vi "Host Approach RetractionA1.vi"() -> ()   [LabVIEW 2012]
uses:
  <vilib>/FPGAPlugInAG/PCI-7831R/niLvFpga_Open_PCI-7831R.vi
  <vilib>/rvi/interface/common/dynamic/niFpgaDynamicAddResources.vi
  <vilib>/Utility/error.llb/Error Cluster From Error Code.vi
  <vilib>/rvi/errors/niLvFpgaAdjustHostInterfaceError.vi
  <vilib>/FPGAPlugInAG/Dynamic/niLvFpga_Close_Dynamic.vi
  <vilib>/FPGAPlugInAG/Dynamic/niLvFpga_Run_Dynamic.vi
  <vilib>/Utility/file.llb/Write To Spreadsheet File (I64).vi
  <vilib>/rvi/interface/nirviOpenFPGA/nirviOpenFPGA.xnode
  SB130-XPS/Documents/FPGA-project-apporach-retraction/FPGA Bitfiles/Apporach-Retract_FPGATarget2_FPGATargetApproa_sPWXUlF8ZuM.lvbitx
  FPGA Target Approach RetractionA2copyAidanV2.vi
  <vilib>/rvi/interface/nirviReadWriteControl/nirviReadWriteControl.xnode
  <vilib>/rvi/interface/nirviCloseFPGA/nirviCloseFPGA.xnode
  <vilib>/rvi/interface/nirviMethod/nirviMethod.xnode
  <vilib>/rvi/interface/Simulation/niFpgaSimulationCallBeginRW.vi
  <vilib>/rvi/errors/niLvFpgaMergeErrorWithErrorCode.vi
  NiFpgaLv.dll
  <vilib>/FPGAPlugInAG/Dynamic/niLvFpga_StartFifo_Dynamic.vi
  <vilib>/FPGAPlugInAG/Dynamic/niLvFpga_StopFifo_Dynamic.vi
  <vilib>/FPGAPlugInAG/Dynamic/niLvFpga_ReadFifo_Dynamic.vi
panel:
  in  "% in for Fast Offset":dbl
  in  "% in for setpoint":dbl
  in  "TF \"Zero\" Point":i16
  out "Bottom Sensor Phase Data":i16[](array[numeric])
  in  "Stop Fine Retraction and start next approach":bool
  in  "Set distance for Bounce or\nretract until TF signal is equal\nto TF in Air":bool
  in  "Bounce Distance (nm)":u32
  out "Fine":i16[](array[numeric])
  out "Course":i16[](array[numeric])
  out "Counter Indicator 2":fxp<+/-,64,32>
  out "fine indicator":i16
  out "TF Phase Data":i16[](graph)
  out "Fine output":i16[](array[numeric])
  out "Course Output":fxp<+/-,64,32>[](array[numeric])
  out "TF Phase data":i16[](array[numeric])
  out "Current Image":u8
  in  "Total Number of Images":u8=1 min=1
  out "step counter":i16
  in  "base path":path=path "C:/Users/Rodolfo/Documents/LAB/2013-05-16-SPM-data"
  in  "file-Name":string="approach-15a"
  in  "Store Data":bool
  out "Bottom Sensor":i16[](graph)
  out "Bottom Sensor \nData":i16[](array[numeric])
  out "Position Data":i16[](array[numeric])
  out "tuning fork amplitude data":i16[](array[numeric])
  in  "Approach Minimum":i32=20000
  out "Approach Setpoint":i32=23000
  out "Fast Approach Offset":i32=29000
  in  "TF in Air":i32=36000
  out "Fine A bits/us":dbl=5.463300000000001e-06
  out "Fine R bits/us":dbl=5.463300000000001e-06
  in  "Fine Approach (nm/s)":dbl=5.0
  in  "Fine Retraction (nm/s)":dbl=5.0
  out "Approach done and fully retracted":bool
  in  "DAQ Rate":i32=8000
  in  "Number of Elements":i32=100
  out "BottomSensor Phase":i16[](graph)
  out "Tuning Fork":i16[](graph)
  out "Fast A nm/s indicator":dbl=200.0
  out "Fast A bits/us":dbl=0.00021853200000000001
  out "Fast R nm/s indicator":dbl=200.0
  out "Fast R bits/us":dbl=0.00021853200000000001
  in  "Fast Approach (nm/s)":dbl=200.0
  in  "Fast Retraction (nm/s)":dbl=200.0
  in  "Automated Approach Start":bool
  out "Numeric":i32=-14468
  out "Counter Indicator":dbl[](graph)
  out "Z Indicator":i16[](graph)
  in  "MCL Counter":i64=100
  in  "MCL Divisions":i32=200
  out "MCL Range Indicator":bool
  out "Host Counter Indicator":i64=115
  out "Digital Steps per Region":i32=327
  out "Host Counter Output":i32=4878
  in  "Z Position MCL Fine":i32
  out "Host Z Position Indicator":i32
  out "Z Position Range Indicator":bool
  out "Z Fine Steps per Region":dbl=0.0049897001602197295
  out "Host Z Output":fxp<+/-,40,30>
  in  "Manual Approach Start":bool
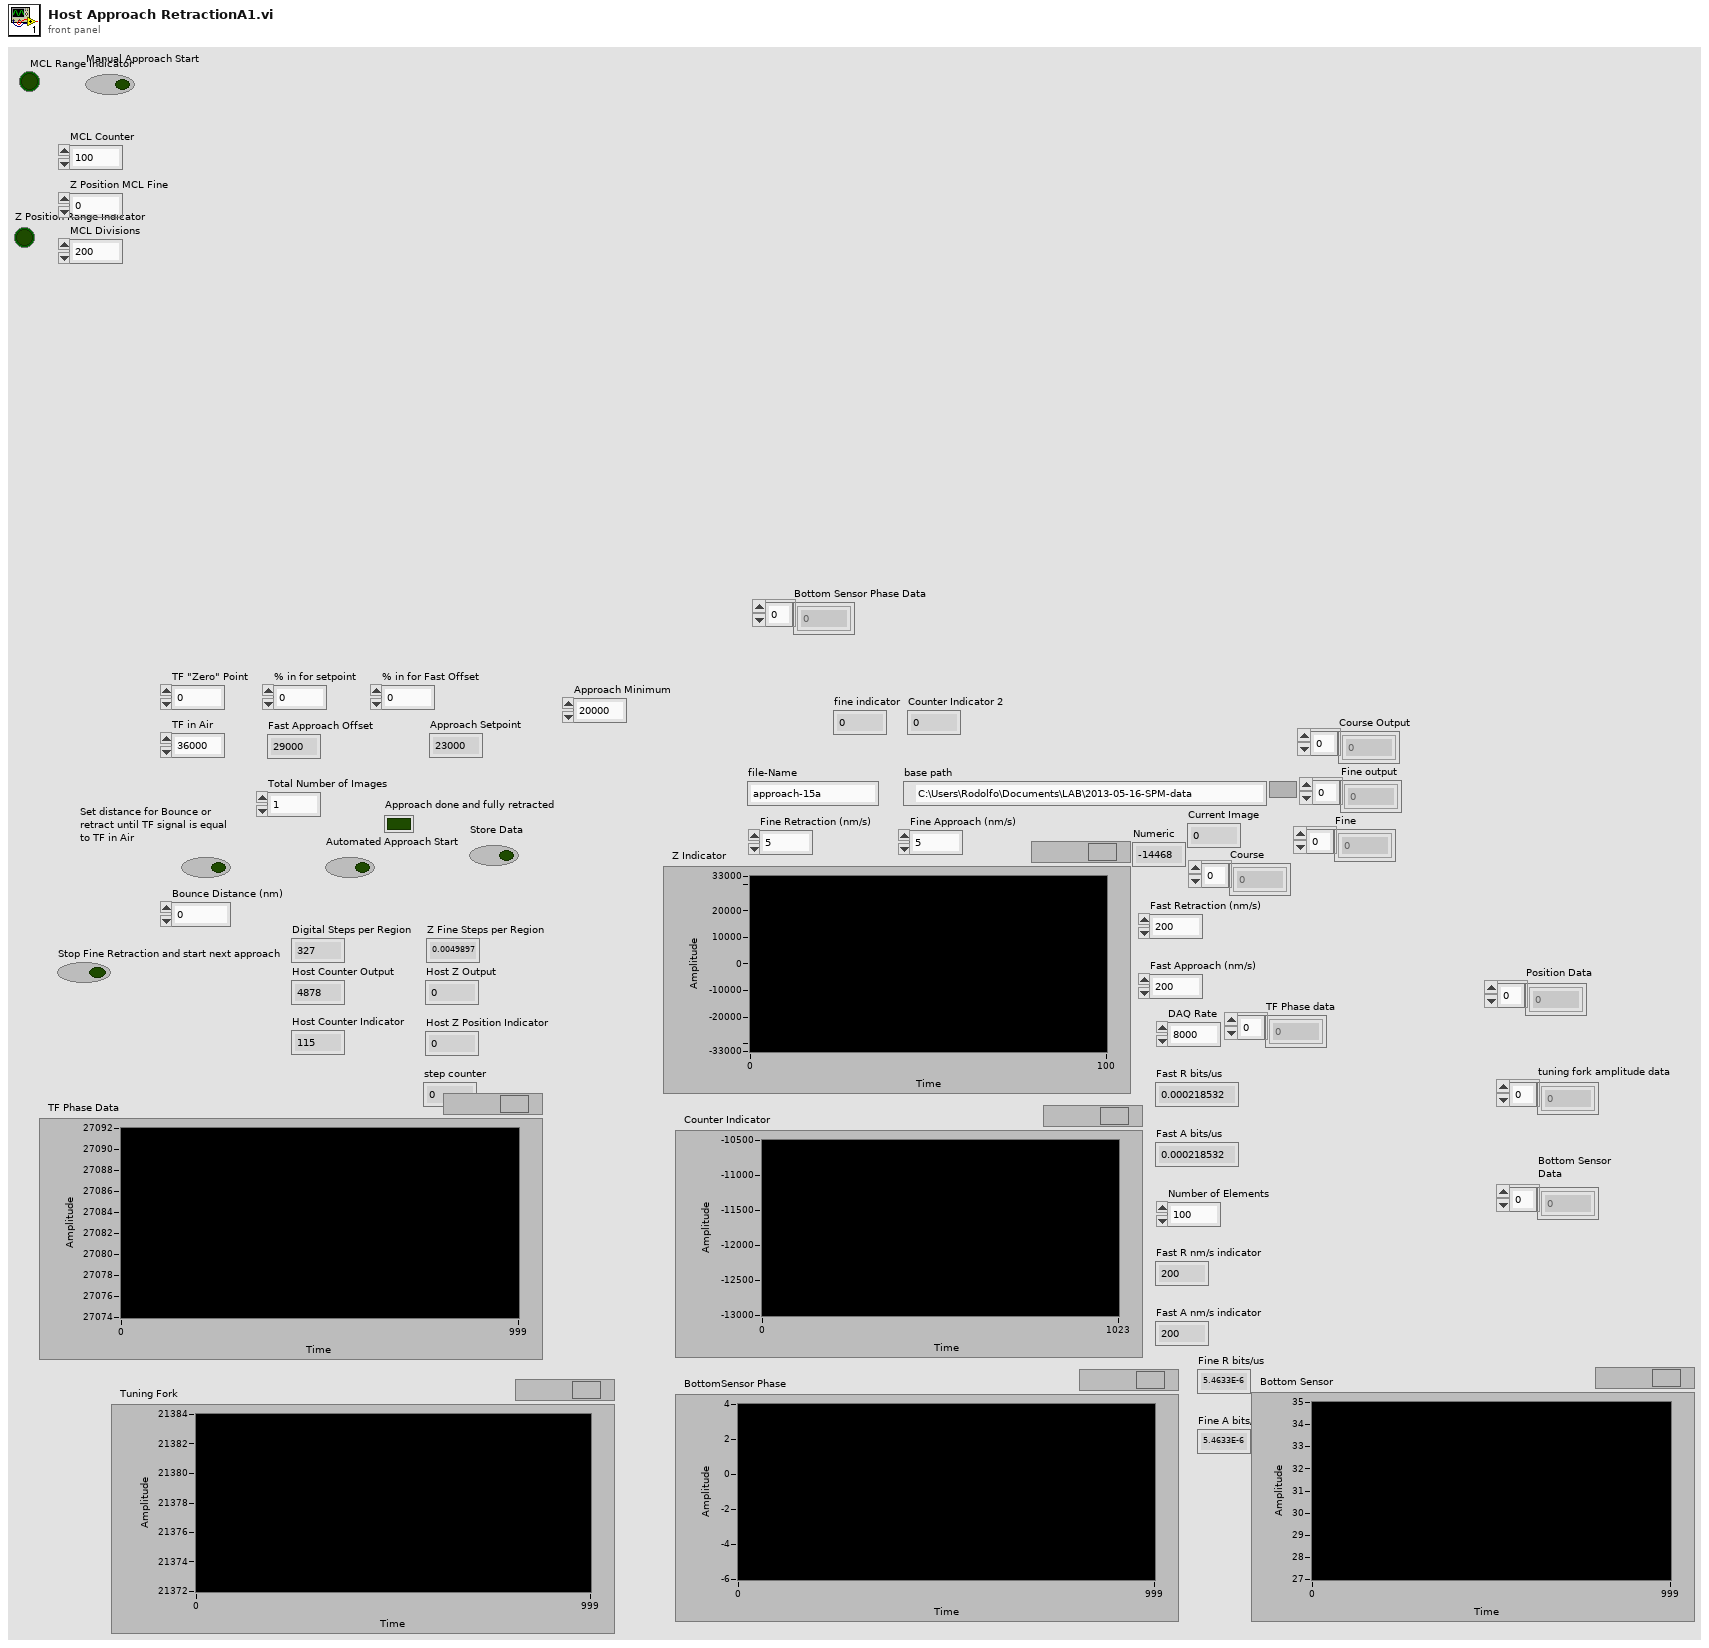
[diagram p1: front panel]
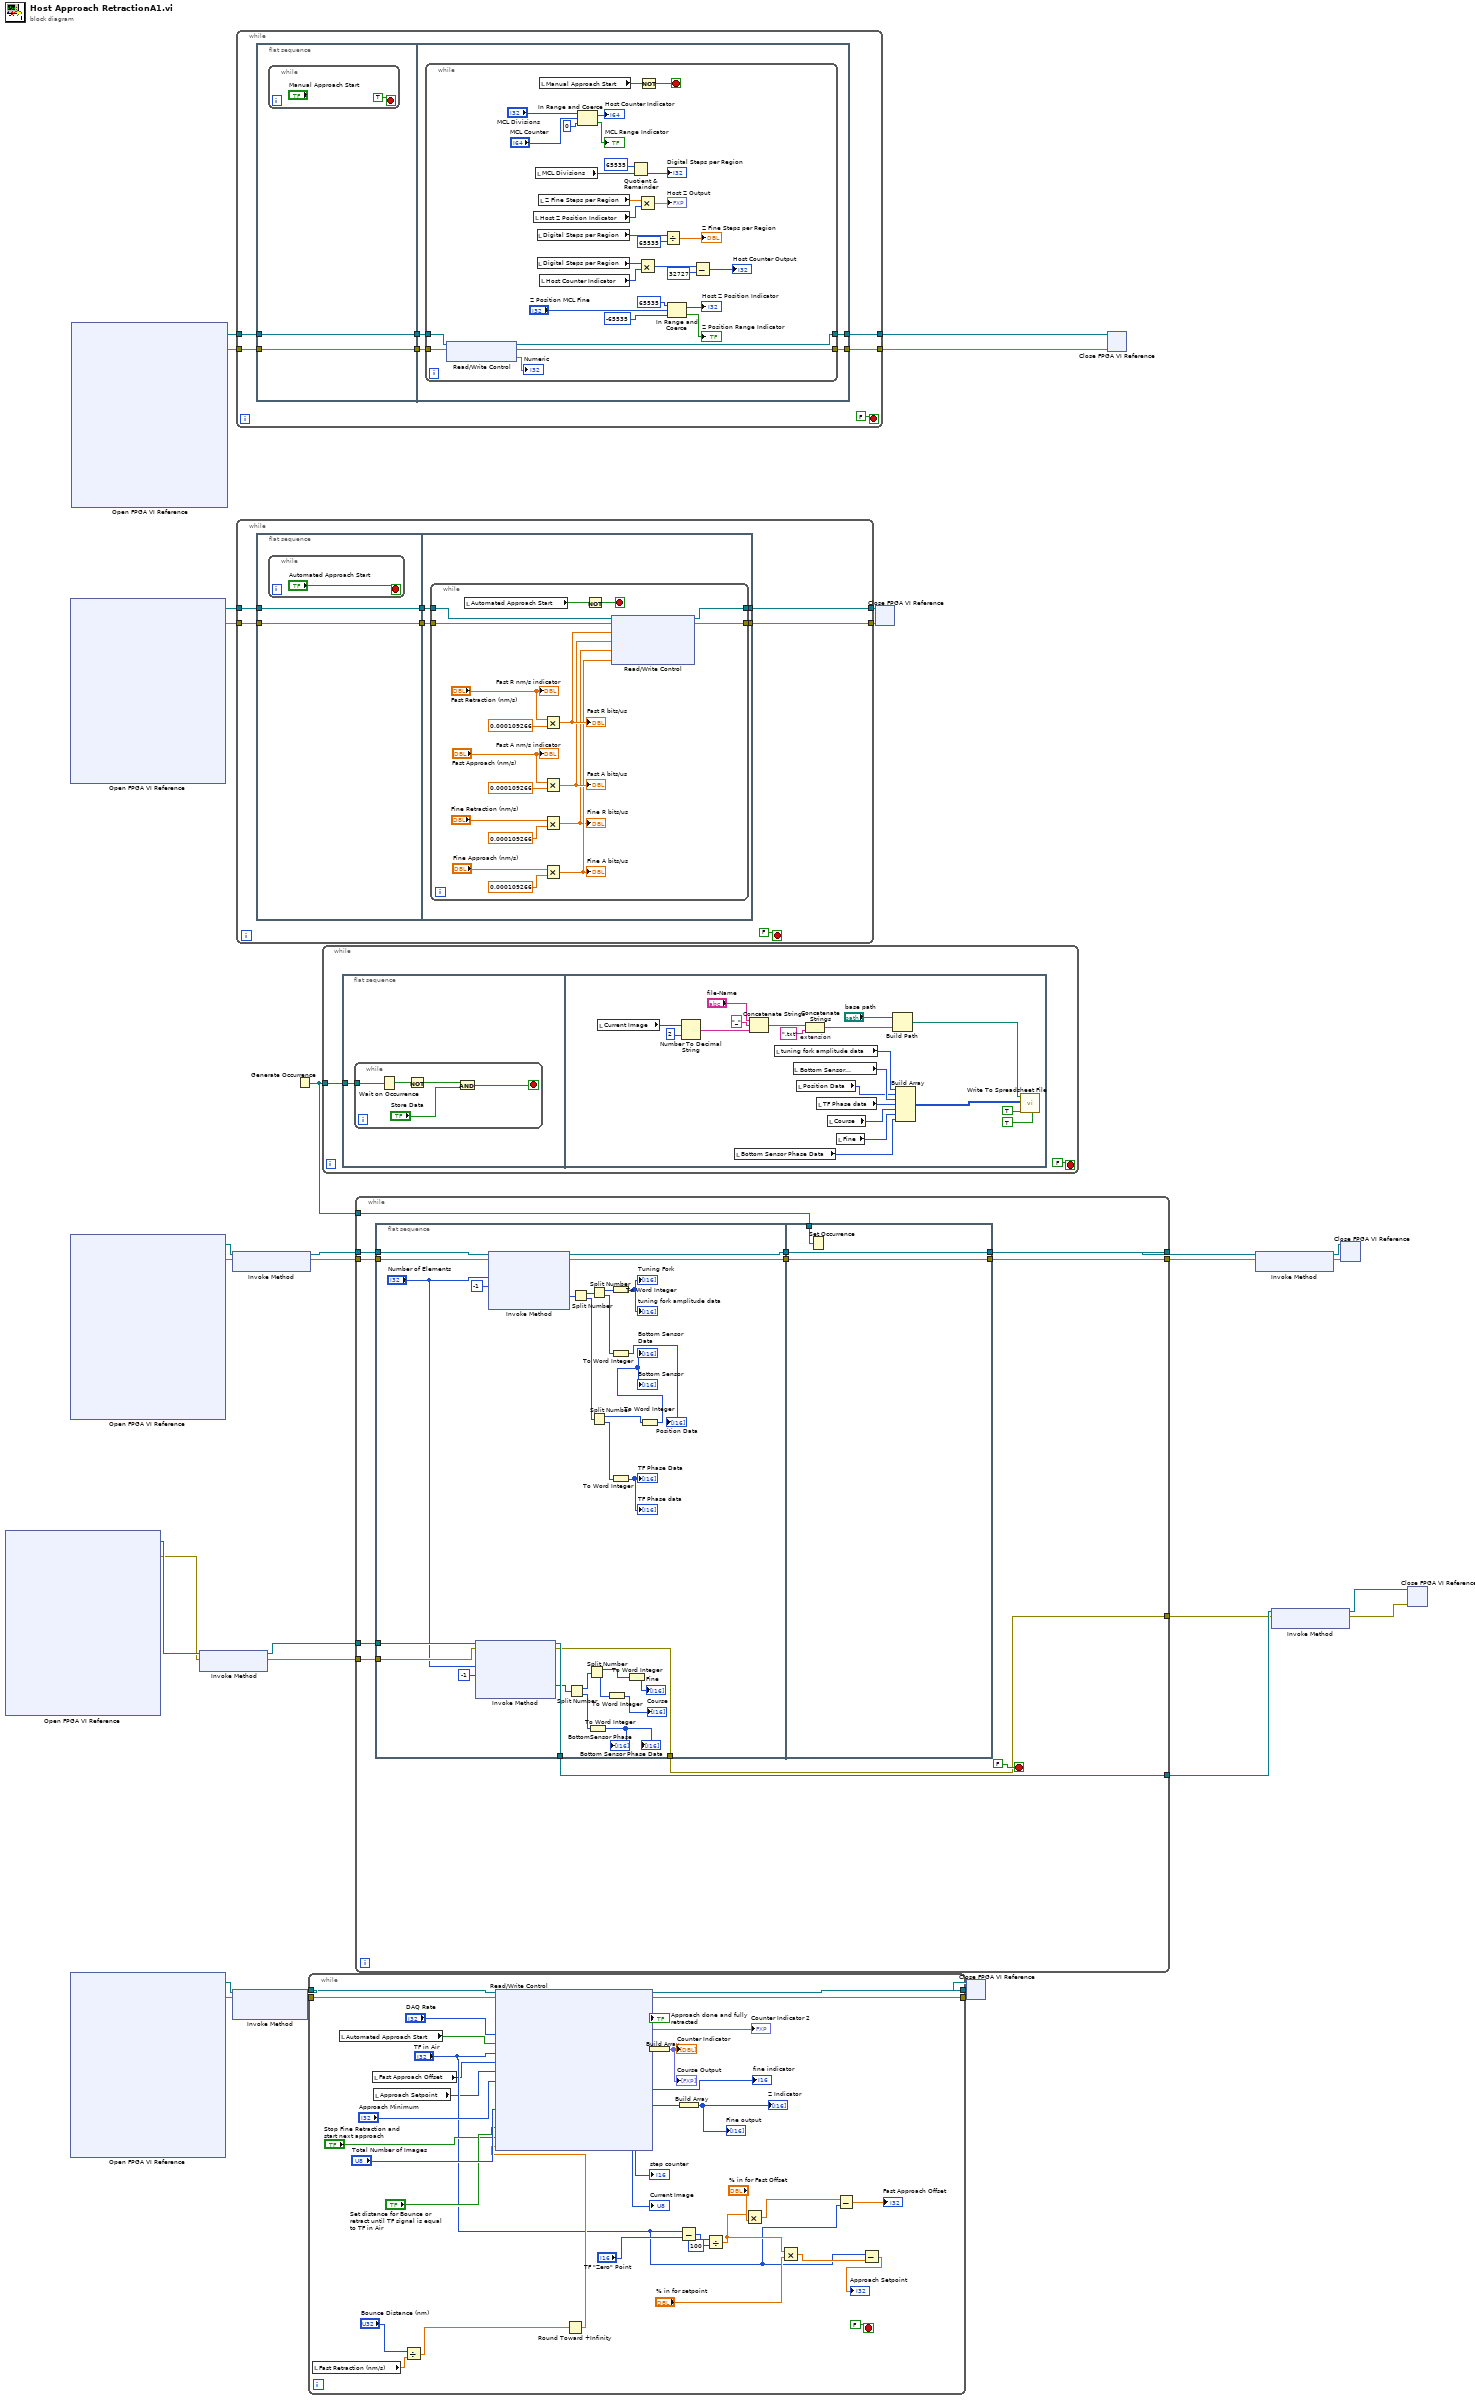
[diagram p0: block diagram]
diagram:
  n1 = xnode "Open FPGA VI Reference"() -> ("FPGA VI Reference Out"=w6:refnum<k20>, "error out"=w5:errorcluster)  [unwired: 2 in]
  n2 = xnode ("Open FPGA VI Reference")() -> ("FPGA VI Reference Out"=w21:refnum<k20>, "error out"=w20:errorcluster)  [unwired: 2 in]
  n3 = xnode "Open FPGA VI Reference"() -> ("FPGA VI Reference Out"=w17:refnum<k20>, "error out"=w16:errorcluster)  [unwired: 2 in]
  n4 = xnode "Open FPGA VI Reference"() -> ("FPGA VI Reference Out"=w23:refnum<k20>, "error out"=w22:errorcluster)  [unwired: 2 in]
  n5 = xnode "Open FPGA VI Reference"() -> ("FPGA VI Reference Out"=w29:refnum<k20>, "error out"=w28:errorcluster)  [unwired: 2 in]
  n6 = xnode "Invoke Method"("FPGA VI Reference In"=w6, "error in"=w5) -> ("FPGA VI Reference Out"=w8:refnum<k20>, "error out"=w7:errorcluster)
  n7 = xnode "Invoke Method"("FPGA VI Reference In"=w17, "error in"=w16) -> ("FPGA VI Reference Out"=w15:refnum<k20>, "error out"=w14:errorcluster)
  n8 = xnode "Invoke Method"("FPGA VI Reference In"=w23, "error in"=w22) -> ("FPGA VI Reference Out"=w25:refnum<k20>, "error out"=w24:errorcluster)  [unwired: 1 in]
  n9 = while {
    tunnel: [w37] -> w31
    tunnel: [w36] -> w30
    tunnel: w29 -> [w34]
    tunnel: w28 -> [w32]
    stop <- FALSE stop-if-true
    n10 = flat-sequence {
      tunnel: [w40] -> w35
      tunnel: w34 -> [w40]
      tunnel: [w39] -> w33
      tunnel: w32 -> [w39]
      tunnel: [w43] -> w37
      tunnel: [w42] -> w36
      tunnel: w35 -> [w45]
      tunnel: w33 -> [w44]
      frame #0 {
        n11 = while {
          stop <- TRUE stop-if-true
        }
      }
      frame #1 {
        n12 = while {
          tunnel: w45 -> [w76]
          tunnel: w44 -> [w75]
          tunnel: [w74] -> w43
          tunnel: [w73] -> w42
          stop <- w71 stop-if-true
          n13 = xnode "Read/Write Control"("FPGA VI Reference In"=w76, "error in"=w75) -> ("FPGA VI Reference Out"=w74:refnum<k20>, "error out"=w73:errorcluster, "Counter Indicator"=→"Numeric":fxp<+/-,64,32>)
          n14 = local read "Host Z Position Indicator"() -> (w48:i32)
          n15 = local read "MCL Divisions"() -> (w64:i32)
          n16 = local read "Digital Steps per Region"() -> (w52:i32)
          n17 = local read "Digital Steps per Region"() -> (w60:i32)
          n18 = local read "Z Fine Steps per Region"() -> (w49:dbl)
          n19 = local read "Manual Approach Start"() -> (w72:bool)
          n20 = local read "Host Counter Indicator"() -> (w59:i64)
          n21 = In Range and Coerce(upper limit="MCL Divisions", x="MCL Counter", lower limit=0) -> (coerced(x)=→"Host Counter Indicator":i64, In Range?=→"MCL Range Indicator":bool)
          n22 = Quotient & Remainder(x=65535, y=w64) -> (floor(x/y)=→"Digital Steps per Region":i32)  [unwired: 1 out]
          n23 = Multiply(x=w49, y=w48) -> (x*y=→"Host Z Output":dbl)
          n24 = Multiply(x=w60, y=w59) -> (x*y=w61:i64)
          n25 = Not(x=w72) -> (.not. x?=w71:bool)
          n26 = Divide(x=w52, y=65535) -> (x/y=→"Z Fine Steps per Region":dbl)
          n27 = In Range and Coerce(upper limit=65535, x="Z Position MCL Fine", lower limit=-65535) -> (coerced(x)=→"Host Z Position Indicator":i32, In Range?=→"Z Position Range Indicator":bool)
          n28 = Subtract(x=w61, y=32727) -> (x-y=→"Host Counter Output":i64)
        }
      }
    }
  }
  n29 = while {
    tunnel: w21 -> [w82]
    tunnel: w20 -> [w81]
    tunnel: [w78] -> w19
    tunnel: [w77] -> w18
    stop <- FALSE stop-if-true
    n30 = flat-sequence {
      tunnel: w82 -> [w85]
      tunnel: w81 -> [w84]
      tunnel: [w85] -> w80
      tunnel: [w84] -> w79
      tunnel: w80 -> [w90]
      tunnel: w79 -> [w89]
      tunnel: [w88] -> w78
      tunnel: [w87] -> w77
      frame #0 {
        n31 = while {
          stop <- "Automated Approach Start" stop-if-true
        }
      }
      frame #1 {
        n32 = while {
          tunnel: w90 -> [w100]
          tunnel: w89 -> [w99]
          tunnel: [w102] -> w88
          tunnel: [w101] -> w87
          stop <- w108 stop-if-true
          n33 = local read "Automated Approach Start"() -> (w107:bool)
          n34 = Multiply(x="Fast Retraction (nm/s)", y=0.000109266) -> (x*y=w98:dbl)
          "Fast R bits/us" <- w98
          n35 = Multiply(x="Fast Approach (nm/s)", y=0.000109266) -> (x*y=w97:dbl)
          "Fast A bits/us" <- w97
          n36 = Multiply(x="Fine Retraction (nm/s)", y=0.000109266) -> (x*y=w91:dbl)
          "Fine R bits/us" <- w91
          n37 = Multiply(x="Fine Approach (nm/s)", y=0.000109266) -> (x*y=w92:dbl)
          "Fine A bits/us" <- w92
          n38 = Not(x=w107) -> (.not. x?=w108:bool)
          n39 = xnode "Read/Write Control"("FPGA VI Reference In"=w100, "error in"=w99, "Fast Retraction Speed"=w98, "Fast Approach Speed"=w97, "Fine Retraction Speed"=w91, "Fine Approach Speed"=w92) -> ("FPGA VI Reference Out"=w102:refnum<k20>, "error out"=w101:errorcluster)
          "Fast R nm/s indicator" <- "Fast Retraction (nm/s)"
          "Fast A nm/s indicator" <- "Fast Approach (nm/s)"
        }
      }
    }
  }
  n40 = Generate Occurrence() -> (w9:refnum<k4>)
  n41 = while {
    tunnel: w25 -> [w142]
    tunnel: w24 -> [w141]
    tunnel: [w140] -> w27
    tunnel: [w139] -> w26
    stop <- FALSE stop-if-true
    n42 = local read "Fast Retraction (nm/s)"() -> (w124:dbl)
    n43 = local read "Automated Approach Start"() -> (w133:bool)
    n44 = local read "Fast Approach Offset"() -> (w110:i32)
    n45 = local read "Approach Setpoint"() -> (w109:i32)
    n46 = Divide(x="Bounce Distance (nm)", y=w124) -> (x/y=w123:dbl)
    n47 = Round Toward +Infinity(x=w123) -> (ceil(x): smallest int >= x=w122:dbl)
    n48 = xnode "Read/Write Control"("FPGA VI Reference In"=w142, "error in"=w141, "Data Acquisition Rate"="DAQ Rate", "Approach"=w133, "TF in Air"="TF in Air", "Fast Approach Offset"=w110, "Approach Setpoint"=w109, "Approach Minimum"="Approach Minimum", "Total Number of Images"="Total Number of Images", "Set \"bounce\" distance or  retract until"="Set distance for Bounce or\nretract until TF signal is equal\nto TF in Air", "Stop Fine Retraction and start next approach"="Stop Fine Retraction and start next approach", "bounce distance control"=w122) -> ("FPGA VI Reference Out"=w140:refnum<k20>, "error out"=w139:errorcluster, "Approaches done and fully retracted"=→"Approach done and fully retracted":bool, "Counter Indicator"=w129:fxp<+/-,64,32>, "fine indicator"=w135:i16, "Step counter"=→"step counter":i16, "Current Image"=→"Current Image":u8)  [unwired: 1 out]
    "fine indicator" <- w135
    "Counter Indicator 2" <- w129
    n49 = Build Array(w129) -> (→"Counter Indicator" →"Course Output":fxp<+/-,64,32>[])
    n50 = Build Array(w135) -> (→"Z Indicator" →"Fine output":i16[])
    n51 = Subtract(x="TF in Air", y="TF \"Zero\" Point") -> (x-y=w120:i32)
    n52 = Divide(x=w120, y=100) -> (x/y=w116:dbl)
    n53 = Multiply(x=w116, y="% in for Fast Offset") -> (x*y=w114:dbl)
    n54 = Multiply(x=w116, y="% in for setpoint") -> (x*y=w115:dbl)
    n55 = Subtract(x=w114, y="TF in Air") -> (x-y=→"Fast Approach Offset":dbl)
    n56 = Subtract(x="TF in Air", y=w115) -> (x-y=→"Approach Setpoint":dbl)
  }
  n57 = while {
    tunnel: w9 -> [w145]
    stop <- FALSE stop-if-true
    n58 = flat-sequence {
      tunnel: w145 -> [w146]
      frame #0 {
        n59 = while {
          tunnel: w146 -> [w151]
          stop <- w147 stop-if-true
          n60 = Wait on Occurrence(2:w151) -> (0:w149:bool)  [unwired: 2 in]
          n61 = Not(x=w149) -> (.not. x?=w148:bool)
          n62 = And(x=w148, y="Store Data") -> (x .and. y?=w147:bool)
        }
      }
      frame #1 {
        n63 = local read "Current Image"() -> (w161:u8)
        n64 = Number To Decimal String(number=w161, width (-)=i16 2) -> (decimal integer string=w159:string)
        n65 = local read "Bottom Sensor Phase Data"() -> (w154:i16[])
        n66 = Concatenate Strings("file-Name", "_", w159) -> (w162:string)
        n67 = local read "tuning fork amplitude data"() -> (w171:i16[])
        n68 = local read "Bottom Sensor \nData"() -> (w153:i16[])
        n69 = local read "Position Data"() -> (w152:i16[])
        n70 = Concatenate Strings "extension"(w162, ".txt" ("string")) -> (w165:string)
        n71 = local read "TF Phase data"() -> (w157:i16[])
        n72 = local read "Course"() -> (w155:i16[])
        n73 = local read "Fine"() -> (w156:i16[])
        n74 = Build Path(base path="base path", name or relative path=w165) -> (appended path=w164:path)
        n75 = Build Array(w171, w152, w153, w157, w155, w156, w154) -> (w170:i16[][])
        n76 = call-poly <vilib>:"Write To Spreadsheet File.vi"("transpose? (no:F)"=TRUE, "append to file? (new file:F)"=TRUE, "2D data"=w170, "file path (dialog if empty)"=w164) -> ()  [unwired: 4 in, 1 out]
      }
    }
  }
  n77 = while {
    tunnel: w15 -> [w183]
    tunnel: w14 -> [w182]
    tunnel: [w181] -> w13
    tunnel: [w180] -> w12
    tunnel: w9 -> [w176]
    tunnel: w8 -> [w175]
    tunnel: w7 -> [w174]
    tunnel: [w173] -> w4
    tunnel: [w172] -> w3
    stop <- FALSE stop-if-true
    n78 = flat-sequence {
      tunnel: w183 -> [w213]
      tunnel: w182 -> [w212]
      tunnel: [w211] -> w178
      tunnel: [w210] -> w177
      tunnel: w175 -> [w199]
      tunnel: w174 -> [w198]
      tunnel: [w197] -> w173
      tunnel: [w196] -> w172
      tunnel: [w215] -> w180
      tunnel: [w216] -> w181
      tunnel: w178 -> [w216]
      tunnel: w177 -> [w215]
      tunnel: w176 -> [w214]
      frame #0 {
        n79 = xnode "Invoke Method"("FPGA VI Reference In"=w199, "error in"=w198, "Number of Elements"="Number of Elements", "Timeout (ms)"=-1) -> ("FPGA VI Reference Out"=w197:refnum<k20>, "error out"=w196:errorcluster, "Data"=w193:i16[])  [unwired: 1 out]
        n80 = xnode "Invoke Method"("FPGA VI Reference In"=w213, "error in"=w212, "Number of Elements"="Number of Elements", "Timeout (ms)"=-1) -> ("FPGA VI Reference Out"=w211:refnum<k20>, "error out"=w210:errorcluster, "Data"=w208:i64[])  [unwired: 1 out]
        n81 = Split Number(x=w193) -> (hi(x)=w191:u8[], lo(x)=w187:u8[])
        n82 = Split Number(x=w208) -> (hi(x)=w207:u32[], lo(x)=w206:u32[])
        n83 = Split Number(x=w191) -> (hi(x)=w189:u8[], lo(x)=w190:u8[])
        n84 = To Word Integer(number=w187) -> (16bit integer=→"BottomSensor Phase" →"Bottom Sensor Phase Data":i16[])
        n85 = Split Number(x=w207) -> (hi(x)=w205:u16[], lo(x)=w203:u16[])
        n86 = Split Number(x=w206) -> (hi(x)=w202:u16[], lo(x)=w201:u16[])
        n87 = To Word Integer(number=w190) -> (16bit integer=→"Course":i16[])
        n88 = To Word Integer(number=w205) -> (16bit integer=→"Tuning Fork" →"tuning fork amplitude data":i16[])
        n89 = To Word Integer(number=w203) -> (16bit integer=→"Position Data":i16[])
        n90 = To Word Integer(number=w201) -> (16bit integer=→"TF Phase data" →"TF Phase Data":i16[])
        n91 = To Word Integer(number=w189) -> (16bit integer=→"Fine":i16[])
        n92 = To Word Integer(number=w202) -> (16bit integer=→"Bottom Sensor" →"Bottom Sensor \nData":i16[])
      }
      frame #1 {
        n93 = Set Occurrence(w214) -> ()
      }
    }
  }
  n94 = xnode "Close FPGA VI Reference"("FPGA VI Reference In"=w19, "error in"=w18) -> ()  [unwired: 1 out]
  n95 = xnode "Close FPGA VI Reference"("FPGA VI Reference In"=w27, "error in"=w26) -> ()  [unwired: 1 out]
  n96 = xnode "Close FPGA VI Reference"("FPGA VI Reference In"=w31, "error in"=w30) -> ()  [unwired: 1 out]
  n97 = xnode "Invoke Method"("FPGA VI Reference In"=w13, "error in"=w12) -> ("FPGA VI Reference Out"=w11:refnum<k20>, "error out"=w10:errorcluster)
  n98 = xnode "Invoke Method"("FPGA VI Reference In"=w4, "error in"=w3) -> ("FPGA VI Reference Out"=w2:refnum<k20>, "error out"=w1:errorcluster)
  n99 = xnode "Close FPGA VI Reference"("FPGA VI Reference In"=w11, "error in"=w10) -> ()  [unwired: 1 out]
  n100 = xnode "Close FPGA VI Reference"("FPGA VI Reference In"=w2, "error in"=w1) -> ()  [unwired: 1 out]
